vi "Physical Memory Monitor.vi"() -> ()   [LabVIEW 2010]
uses:
  kernel32.dll
panel:
  in  "Close":bool
  out "error out":errorcluster
  out "Total":dbl
  out "Available":dbl
  out "Free memory (%)":dbl
  out "Memory Usage":dbl(slide) scale=0.0..100.0
  out "Memory Usage History":dbl(graph)
  # "QIG-IPG Tester"
  # "Memory Monitor"
  # "Available Memory"
  # "Memory Usage"
  # "Physical Memory (MB)"
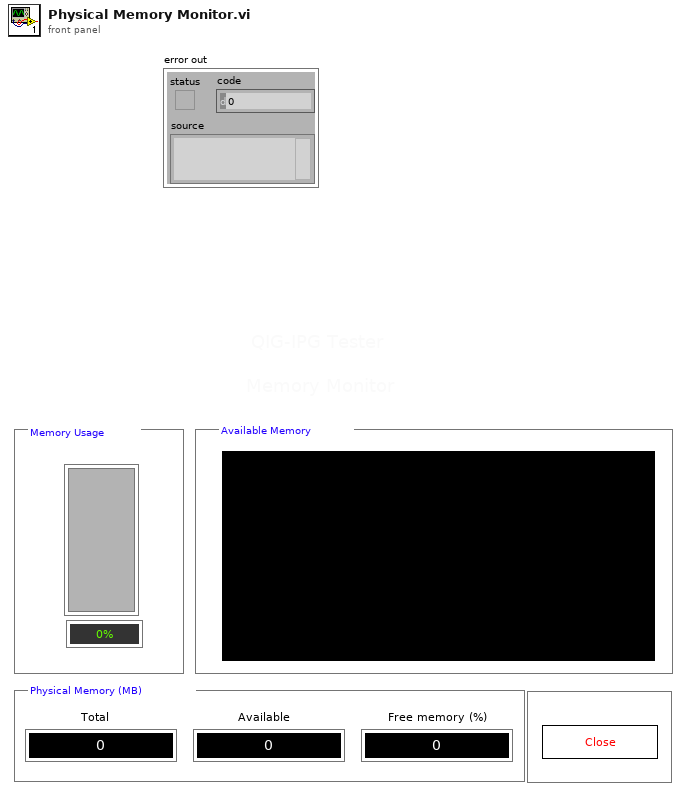
[diagram p1: front panel]
types:
  T1 = cluster{"dwLength":u32, "dwMemoryLoad":u32, "ullTotalPhys":u64, "ullAvailPhys":u64, "ullTotalPageFile":u64, "ullAvailPageFile":u64, "ullTotalVirtual":u64, "ullAvailVirtual":u64, "ullAvailExtendedVirtual":u64}
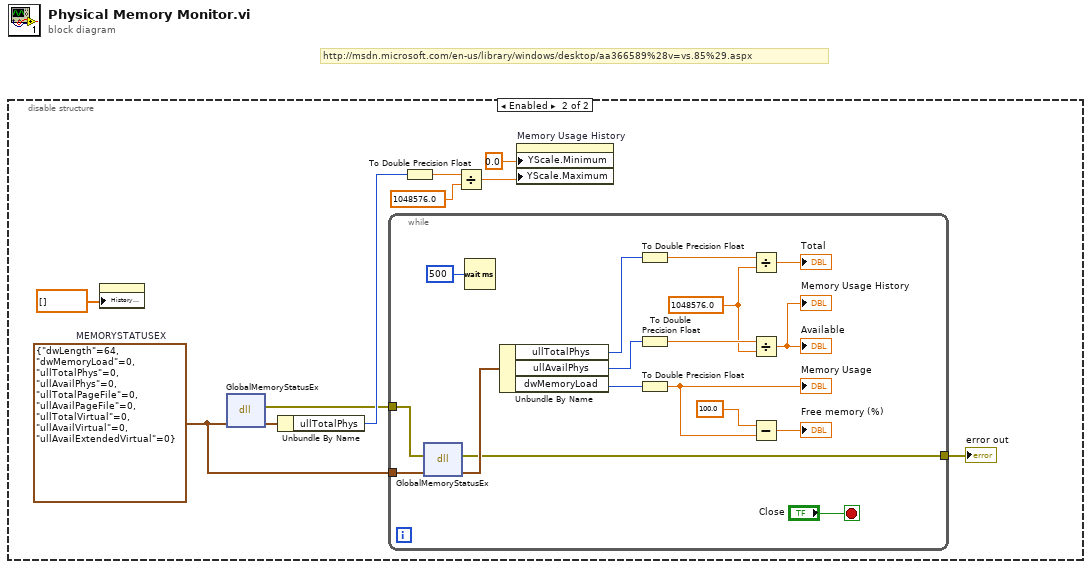
[diagram p0: block diagram]
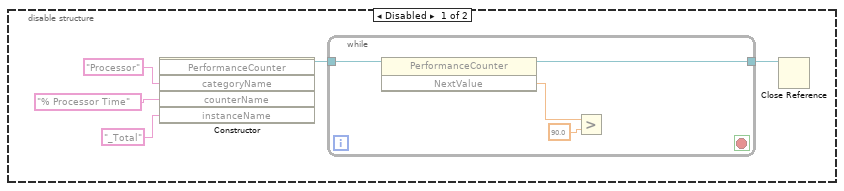
[diagram p2: hidden frame]
diagram:
  # "http://msdn.microsoft.com/en-us/library/windows/desktop/aa366589%28v=vs.85%29.aspx"
  n1 = disable-structure shown="Enabled" {
    frame Disabled {
      n2 = constructor class="PerformanceCounter"("categoryName"="Processor", "counterName"="% Processor Time", "instanceName"="_Total") -> (reference out=w2:refnum<k24>)  [unwired: 3 in, 5 out]
      n3 = while {
        tunnel: w2 -> [w9]
        tunnel: [w8] -> w1
        stop <- _ stop-if-true
        n4 = invoke class="PerformanceCounter" method="NextValue"(reference=w9) -> (reference out=w8:refnum<k24>, "NextValue"=w7:sgl)  [unwired: 2 in, 1 out]
        n5 = Greater?(x=w7, y=sgl 90.0) -> ()  [unwired: 1 out]
      }
      n6 = Close Reference(reference=w1) -> ()  [unwired: 1 in, 1 out]
    }
    frame Enabled {
      w17 = T1 {"dwLength"=64, "dwMemoryLoad"=0, "ullTotalPhys"=0, "ullAvailPhys"=0, "ullTotalPageFile"=0, "ullAvailPageFile"=0, "ullTotalVirtual"=0, "ullAvailVirtual"=0, "ullAvailExtendedVirtual"=0}  # MEMORYSTATUSEX
      n7 = property on="Memory Usage History" class="WFChart (strict)"("History Data"=dbl[] []) -> ()  [unwired: 2 in, 2 out]
      n8 = dll-call lib="kernel32.dll" fn="GlobalMemoryStatusEx"(w17) -> (error out=w11:errorcluster, w13:T1)  [unwired: 4 in, 1 out]
      n9 = Unbundle By Name(w13) -> ("ullTotalPhys"=w16:u64)
      n10 = while {
        tunnel: w17 -> [w30]
        tunnel: w11 -> [w22]
        tunnel: [w21] -> w10
        stop <- "Close" stop-if-true
        w32 = 1048576.0 ("y")
        n11 = dll-call lib="kernel32.dll" fn="GlobalMemoryStatusEx"(error in=w22, w30) -> (error out=w21:errorcluster, w29:T1)  [unwired: 3 in, 1 out]
        n12 = Wait (ms)(milliseconds to wait=u32 500) -> ()  [unwired: 1 out]
        n13 = Unbundle By Name(w29) -> ("ullTotalPhys"=w36:u64, "ullAvailPhys"=w34:u64, "dwMemoryLoad"=w26:u32)
        n14 = To Double Precision Float(number=w36) -> (double precision float=w35:dbl)
        n15 = To Double Precision Float(number=w34) -> (double precision float=w33:dbl)
        n16 = To Double Precision Float(number=w26) -> (double precision float=w24:dbl)
        "Memory Usage" <- w24
        n17 = Divide(x=w35, y=w32) -> (x/y=→"Total":dbl)
        n18 = Divide(x=w33, y=w32) -> (x/y=→"Available" →"Memory Usage History":dbl)
        n19 = Subtract(x=100.0, y=w24) -> (x-y=→"Free memory (%)":dbl)
      }
      "error out" <- w10
      n20 = To Double Precision Float(number=w16) -> (double precision float=w15:dbl)
      n21 = Divide(x=w15, y=1048576.0) -> (x/y=w18:dbl)
      n22 = property on="Memory Usage History" class="WFChart (strict)"("YScale.Minimum"=0.0 ("Y Scale.Range:Minimum"), "YScale.Maximum"=w18) -> ()  [unwired: 2 in, 2 out]
    }
  }
